vi "Falling Edge (T init).vi"(5 "Signal":bool) -> (2 "Edge Detected":bool)   [LabVIEW 2021, in "Boolean_CIF_U.lvlib"]
uses:
  Boolean_CIF_U.lvlib
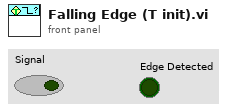
[diagram p1: front panel]
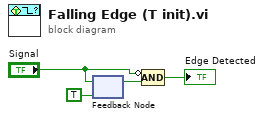
[diagram p0: block diagram]
diagram:
  n1 = feedback #1(TRUE) -> (w3:bool)
  n2 = feedback-in #1("Signal") -> ()
  n3 = Compound Arithmetic op=AND(invert "Signal", w3) -> (→"Edge Detected":bool)
